vi "GPS_Xy.vi"(10 "Log Data In":cluster{refnum<class "RDS State.lvclass">[]}[](array[cluster]), 11 "Log Header":T1) -> (2 "Log Data Out":cluster{refnum<class "RDS State.lvclass">[]}[](array[cluster]), 3 "Log Header Out":T1, 5 "Lat Long":T2(array[cluster]))   [LabVIEW 2015, in "Log Waveform Processors.lvlib"]
uses:
  Log Waveform Processors.lvlib
  RDS State Tracker/RDS State/RDS State.lvclass
  Actors/RDS Logger Actor/RDS Logger Actor/RDS Logger Actor/Logger Header.ctl
  RDS State Tracker/RDS State/RDS State.lvclass/RDS State.ctl
  <vilib>/measure/maresamp.llb/Resample Waveform (single shot).vi
  <vilib>/measure/NI_MAPro.lvlib
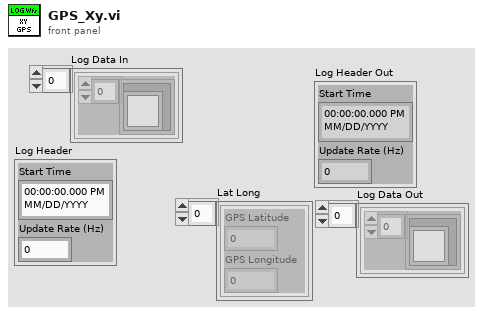
[diagram p1: front panel]
types:
  T1 = typedef "Log Waveform Processors.lvlib/Logger Header.ctl" = cluster{"Start Time":timestamp, "Update Rate (Hz)":dbl}
  T2 = cluster{"GPS Latitude":ext, "GPS Longitude":ext}[]
  T3 = typedef "RDS Libraries.lvlib/NMEA.lvlib/NMEA_GPRMC-data.ctl" = cluster{"TimeStamp":timestamp, "Validity":bool, "Latitude":dbl, "Latitude-Direction":T4, "Longitude":dbl, "Longitude-Direction":T5, "Speed in knots":sgl, "True course":sgl, "Date Stamp":timestamp, "Magnetic Variation (East/West)":sgl, "GPS Latitude":dbl, "GPS Longitude":dbl}
  T4 = typedef "RDS Libraries.lvlib/NMEA.lvlib/NMEA_LatitudeDirection.ctl" = enum16{"", "North", "South"}
  T5 = typedef "RDS Libraries.lvlib/NMEA.lvlib/NMEA_LongitudeDirection.ctl" = enum16{"", "East", "West"}
  T6 = typedef "RDS Instrument Library.lvlib/Compass Data.ctl" = cluster{"Compass Heading":sgl, "pitch Angle":sgl, "roll Angle":sgl, "Temperature":sgl, "Depth":sgl, "Magnetic Field":sgl, "Magnetic Field X":sgl, "Magnetic Field Y":sgl, "Magnetic Field Z":sgl, "Acceleration":sgl, "Acceleration X":sgl, "Acceleration Y":sgl, "Gyro":sgl, "Gyro X":sgl, "Acceleration Z":sgl, "Gyro Y":sgl, "Raw Heading":sgl}
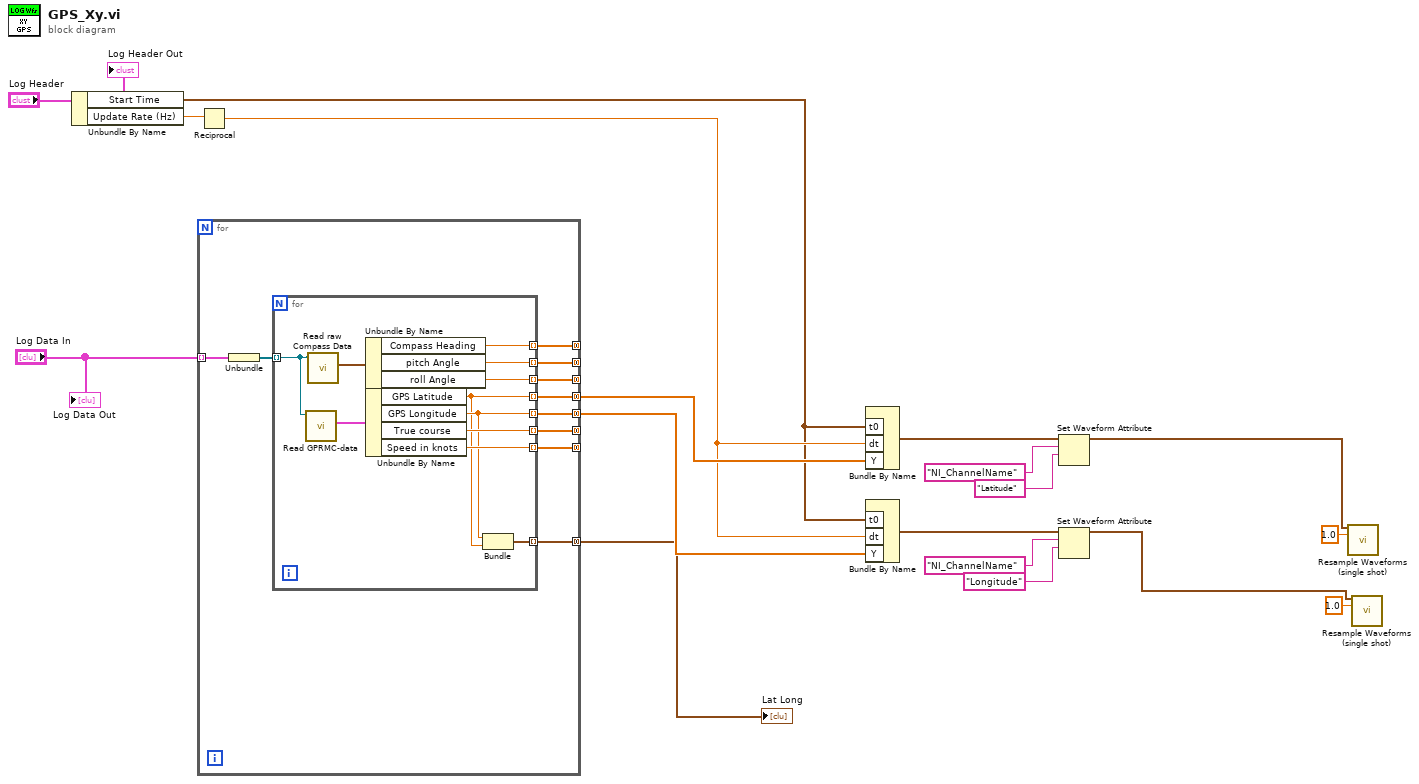
[diagram p0: block diagram]
diagram:
  n1 = Unbundle By Name("Log Header") -> ("Start Time"=w2:timestamp, "Update Rate (Hz)"=w8:dbl)
  n2 = for {
    tunnel: "Log Data In" -> [w28] mode=indexing
    tunnel: [w26] -> _ mode=concatenating
    tunnel: [w25] -> _ mode=concatenating
    tunnel: [w24] -> _ mode=concatenating
    tunnel: [w23] -> w17 mode=concatenating
    tunnel: [w22] -> w18 mode=concatenating
    tunnel: [w21] -> _ mode=concatenating
    tunnel: [w20] -> _ mode=concatenating
    tunnel: [w19] -> w1 mode=concatenating
    n3 = Unbundle(w28) -> (w27:refnum<class "RDS State.lvclass">[])
    n4 = for {
      tunnel: w27 -> [w33] mode=indexing
      tunnel: [w39] -> w26 mode=indexing
      tunnel: [w38] -> w25 mode=indexing
      tunnel: [w37] -> w24 mode=indexing
      tunnel: [w30] -> w23 mode=indexing
      tunnel: [w31] -> w22 mode=indexing
      tunnel: [w35] -> w21 mode=indexing
      tunnel: [w34] -> w20 mode=indexing
      tunnel: [w32] -> w19 mode=indexing
      n5 = call "Read GPRMC-data.vi"("RDS State in"=w33) -> ("GPRMC-data"=w29:T3)  [unwired: 8 in, 2 out]
      n6 = call "Read raw Compass Data.vi"("RDS State in"=w33) -> ("Compass Data"=w36:T6)  [unwired: 8 in, 2 out]
      n7 = Unbundle By Name(w36) -> ("Compass Heading"=w39:sgl, "pitch Angle"=w38:sgl, "roll Angle"=w37:sgl)
      n8 = Unbundle By Name(w29) -> ("GPS Latitude"=w30:dbl, "GPS Longitude"=w31:dbl, "True course"=w35:sgl, "Speed in knots"=w34:sgl)
      n9 = Bundle("GPS Longitude"=w31, "GPS Latitude"=w30) -> (w32:cluster{"GPS Longitude":dbl, "GPS Latitude":dbl})  [unwired: 1 in]
    }
  }
  "Lat Long" <- w1
  n10 = Reciprocal(x=w8) -> (1/x=w7:dbl)
  n11 = Bundle By Name("t0"=w2, "dt"=w7, "Y"=w17) -> (w13:waveform(dbl))  [unwired: 1 in]
  n12 = Bundle By Name("t0"=w2, "dt"=w7, "Y"=w18) -> (w14:waveform(dbl))  [unwired: 1 in]
  n13 = Set Waveform Attribute(5:"Latitude" ("name"), 6:"NI_ChannelName" ("name"), 7:w13) -> (3:w6:waveform(dbl))  [unwired: 1 in, 2 out]
  n14 = Set Waveform Attribute(5:"Longitude" ("name"), 6:"NI_ChannelName" ("name"), 7:w14) -> (3:w3:waveform(dbl))  [unwired: 1 in, 2 out]
  n15 = call-poly <vilib>:"Resample Waveforms (single shot).vi"("waveform in"=w6, "dt"=1.0) -> ()  [unwired: 10 in, 4 out]
  n16 = call-poly <vilib>:"Resample Waveforms (single shot).vi"("waveform in"=w3, "dt"=1.0) -> ()  [unwired: 10 in, 4 out]
  "Log Header Out" <- "Log Header"
  "Log Data Out" <- "Log Data In"
